vi "AlarmHandle.vi"(9 "Value":bool, 10 "DigitalAlarmSettings":T2, 11 "AlarmStatus in":T1) -> (3 "AlarmStatus out":T1)   [LabVIEW 2019]
uses:
  TypeDef/CommonAlarmSettings.ctl
  TypeDef/CommonAlarmStatus.ctl
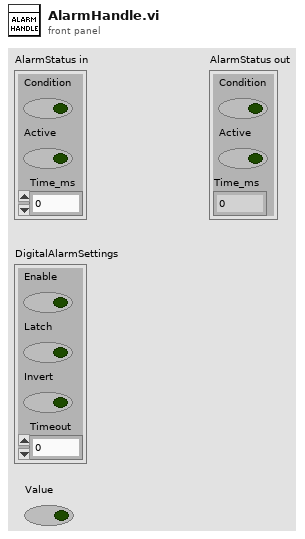
[diagram p1: front panel]
types:
  T1 = typedef "CommonAlarmStatus.ctl" = cluster{"Condition":bool, "Active":bool, "Time_ms":u32}
  T2 = typedef "CommonAlarmSettings.ctl" = cluster{"Enable":bool, "Latch":bool, "Invert":bool, "Timeout":u32}
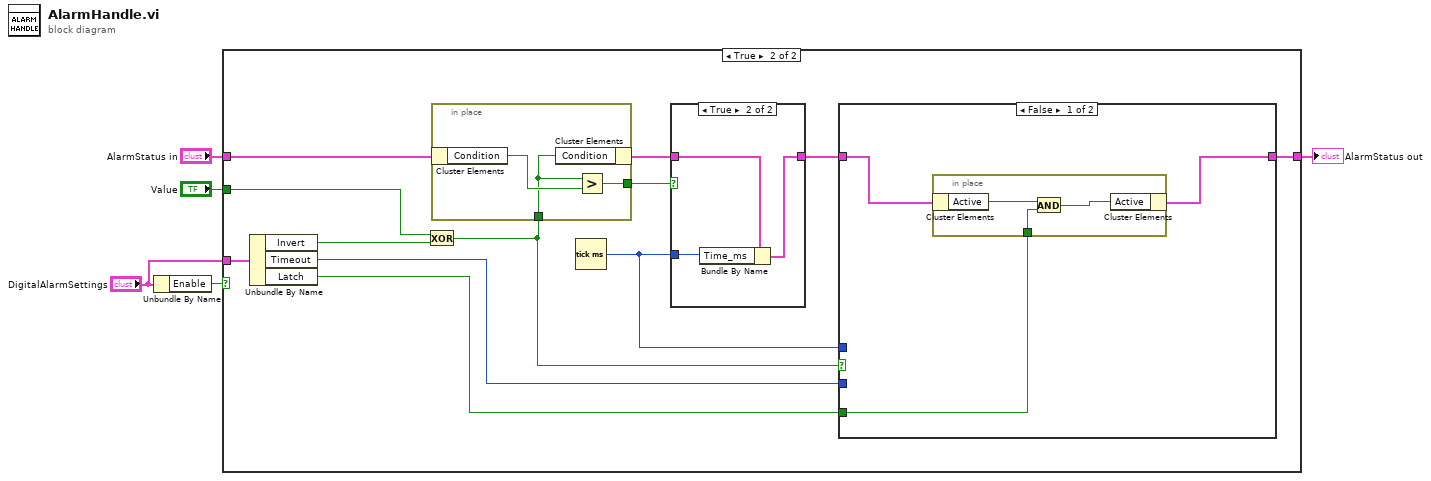
[diagram p0: block diagram]
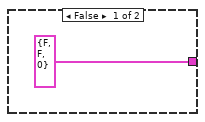
[diagram p2: hidden frame]
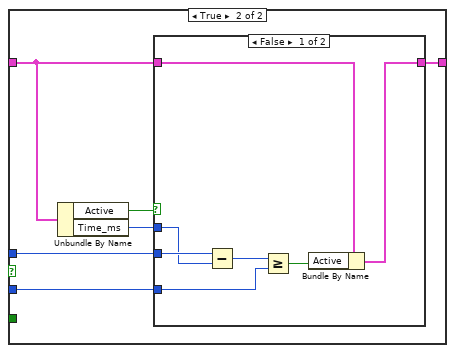
[diagram p3: hidden frame]
diagram:
  n1 = Unbundle By Name("DigitalAlarmSettings") -> ("Enable"=w5:bool)
  n2 = case shown="True" w5 {
    tunnel: "AlarmStatus in" -> [_ w7]
    tunnel: [T1 {"Condition"=FALSE, "Active"=FALSE, "Time_ms"=0} ("AlarmStatus out") w11] -> w3
    tunnel: "Value" -> [_ w16]
    tunnel: "DigitalAlarmSettings" -> [_ w18]
    frame False {
    }
    frame True {
      n3 = Unbundle By Name(w18) -> ("Invert"=w17:bool, "Timeout"=w12:u32, "Latch"=w10:bool)
      n4 = Exclusive Or(1:w17, 2:w16) -> (0:w8:bool)
      n5 = in-place {
        in-place-border: [w41] -> w15
        in-place-border: w8 -> [w39]
        n6 = in-place-cluster #1(w7) -> ("Condition"=w40:bool)
        n7 = in-place-cluster #1("Condition"=w39) -> (w9:T1)
        n8 = Greater?(x=w39, y=w40) -> (0:w41:bool)
      }
      n9 = Tick Count (ms)() -> (millisecond timer value=w13:u32)
      n10 = case shown="True" w15 {
        tunnel: w9 -> [w42 w45]
        tunnel: [w42 w44] -> w14
        tunnel: w13 -> [_ w43]
        frame False {
        }
        frame True {
          n11 = Bundle By Name(cluster=w45, "Time_ms"=w43) -> (w44:T1)
        }
      }
      n12 = case shown="False" w8 {
        tunnel: w14 -> [w21 w27]
        tunnel: w13 -> [_ w30]
        tunnel: w12 -> [_ w28]
        tunnel: [w19 w26] -> w11
        tunnel: w10 -> [w20 _]
        frame False {
          n13 = in-place {
            in-place-border: w20 -> [w23]
            n14 = in-place-cluster #2(w21) -> ("Active"=w24:bool)
            n15 = And(x=w24, y=w23) -> (x .and. y?=w22:bool)
            n16 = in-place-cluster #2("Active"=w22) -> (w19:T1)
          }
        }
        frame True {
          n17 = Unbundle By Name(w27) -> ("Active"=w25:bool, "Time_ms"=w29:u32)
          n18 = case shown="False" w25 {
            tunnel: w30 -> [w37 _]
            tunnel: w29 -> [w36 _]
            tunnel: w28 -> [w34 _]
            tunnel: w27 -> [w33 w38]
            tunnel: [w31 w38] -> w26
            frame False {
              n19 = Subtract(x=w37, y=w36) -> (x-y=w35:u32)
              n20 = Greater Or Equal?(x=w35, y=w34) -> (x >= y?=w32:bool)
              n21 = Bundle By Name(cluster=w33, "Active"=w32) -> (w31:T1)
            }
            frame True {
            }
          }
        }
      }
    }
  }
  "AlarmStatus out" <- w3
